vi "NextDieMove.vi"() -> ()   [LabVIEW 2015]
uses:
  Interface.ctl
panel:
  in  "Interface":T1
  out "NoMoreDieCanMove":bool
  in  "Next/Previous Die":bool
  out "IsAtFinialDie":bool
  out "error code":i32
  out "StringOutputArray":string[](array[string])
  out "Response":string
  in  "VISA Resource":refnum<visa-resource-name>="GPIB0::13::INSTR"
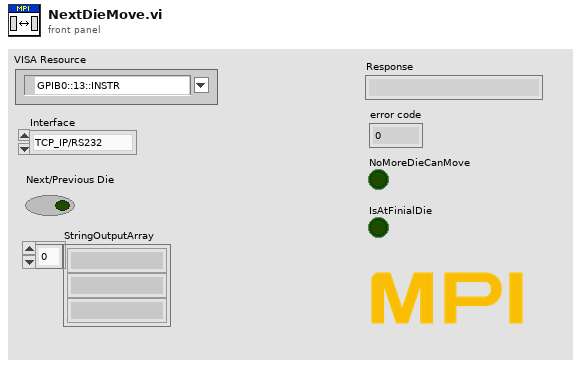
[diagram p1: front panel]
types:
  T1 = typedef "Interface.ctl" = enum16{"TCP_IP/RS232", "GPIB"}
  T2 = enum16{"EndOfLine", "LineFeed", "CarriageReturn"}
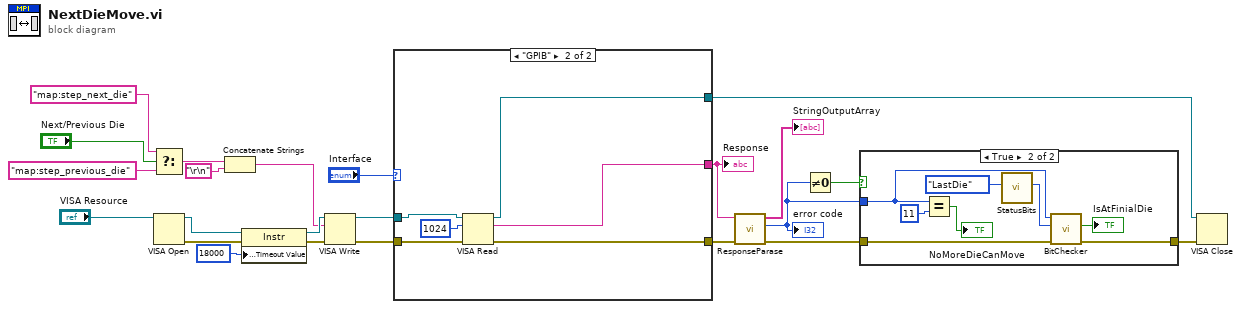
[diagram p0: block diagram]
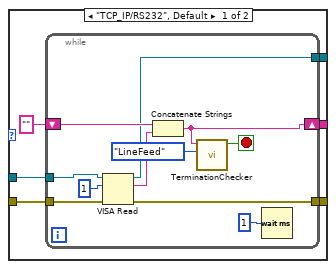
[diagram p2: hidden frame]
diagram:
  n1 = Select(t="map:step_next_die", s="Next/Previous Die", f="map:step_previous_die") -> (s? t:f=w10:string)
  n2 = VISA Open(VISA resource name="VISA Resource") -> (VISA resource name=w21:refnum<visa-resource-name>, error out=w20:errorcluster)  [unwired: 1 in, 3 out]
  n3 = Concatenate Strings(w10, "\r\n") -> (w16:string)
  n4 = property class="Instr"(reference=w21, error in=w20, "General Settings:Timeout Value"=u32 18000) -> (reference out=w19:refnum<visa-resource-name>, error out=w18:errorcluster)
  n5 = VISA Write(VISA resource name=w19, write buffer=w16, error in (no error)=w18) -> (VISA resource name out=w15:refnum<visa-resource-name>, error out=w14:errorcluster)  [unwired: 1 out]
  n6 = case shown="\"GPIB\"" "Interface" {
    tunnel: w15 -> [w29 w45]
    tunnel: w14 -> [w28 w44]
    tunnel: [w26 w41] -> w13
    tunnel: [w25 w43] -> w7
    tunnel: [w24 w42] -> w4
    frame "TCP_IP/RS232", Default {
      n7 = while {
        tunnel: w29 -> [w40]
        tunnel: w28 -> [w39]
        shift-right: [w33] -> w26
        shift-left: "" -> [w37]
        tunnel: [w31] -> w24
        tunnel: [w30] -> w25
        stop <- w35 stop-if-true
        n8 = VISA Read(VISA resource name=w40, byte count=u32 1, error in (no error)=w39) -> (VISA resource name out=w31:refnum<visa-resource-name>, read buffer=w36:string, error out=w30:errorcluster)  [unwired: 1 out]
        n9 = Concatenate Strings(w37, w36) -> (w33:string)
        n10 = call "TerminationChecker.vi"("Type"=T2."LineFeed", "input string"=w33) -> ("Ret"=w35:bool)  [unwired: 9 in]
        n11 = Wait (ms)(milliseconds to wait=u32 1) -> ()  [unwired: 1 out]
      }
    }
    frame "GPIB" {
      n12 = VISA Read(VISA resource name=w45, byte count=u32 1024, error in (no error)=w44) -> (VISA resource name out=w42:refnum<visa-resource-name>, read buffer=w41:string, error out=w43:errorcluster)  [unwired: 1 out]
    }
  }
  "Response" <- w13
  n13 = call "ResponseParase.vi"("error in (no error)"=w7, "input string"=w13) -> ("error out"=w6:errorcluster, "error code"=w2:i32, "OutputArray"=→"StringOutputArray":string[])  [unwired: 7 in]
  "error code" <- w2
  n14 = Not Equal To 0?(x=w2) -> (x != 0?=w3:bool)
  n15 = case shown="True" w3 {
    tunnel: w2 -> [_ w50]
    tunnel: w6 -> [w47 w52]
    tunnel: [w47 w51] -> w5
    frame False {
    }
    frame True {
      n16 = Equal?(x=w50, y=11) -> (x = y?=→"NoMoreDieCanMove":bool)
      n17 = call "StatusBits.vi"("StatusBit"=enum16{"LastSubsite", "LastDie"}."LastDie") -> ("StatusBits"=w53:i32)  [unwired: 10 in]
      n18 = call "BitChecker.vi"("error in (no error)"=w52, "Bit(0-31)"=w53, "Input"=w50) -> ("error out"=w51:errorcluster, "IsSet"=→"IsAtFinialDie":bool)  [unwired: 6 in, 1 out]
    }
  }
  n19 = VISA Close(VISA resource name=w4, error in (no error)=w5) -> ()  [unwired: 1 out]
